vi "Linkages NodeID to GUID.vi"(7 "Response Refnum in":T1 format="%.0x", 8 "error in (no error)":errorcluster, 11 "Linked Channels in":T2[](array[typedef]) {"Channel Refnum" format="%.0x"}) -> (0 "error out":errorcluster, 3 "Linked Channels out":cluster{"Variable Name":string, "GUID":string}[](array[cluster]))   [LabVIEW 2018, in "Instrument Addon Scripting API.lvlib"]
uses:
  Instrument Addon Scripting API.lvlib
  TypeDefs/Linked Channel.ctl
  <vilib>/NI Veristand/Custom Device API/Custom Device Item Ref.ctl
  <vilib>/NI/NI VeriStand Advanced SysDef API/_SubVIs/SysDef.Search.Parent.vi
  Addon/Addon Shared/SubVIs/Constants.vi
  <vilib>/NI Veristand/Custom Device API/Get Item Property (String).vi
  <vilib>/NI Veristand/Custom Device API/Custom Device API.lvlib
  Addon/Addon Shared/Instrument Addon Shared.lvlib
  <vilib>/NI/NI VeriStand Advanced SysDef API/SysDef API/Advanced System Definition.lvlib
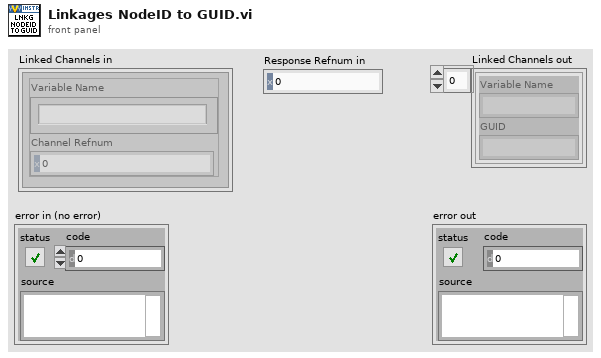
[diagram p1: front panel]
types:
  T1 = typedef "Custom Device API.lvlib/Custom Device Item Ref.ctl" = u64
  T2 = typedef "Instrument Addon Scripting API.lvlib/Linked Channel.ctl" = cluster{"Variable Name":string, "Channel Refnum":T1}
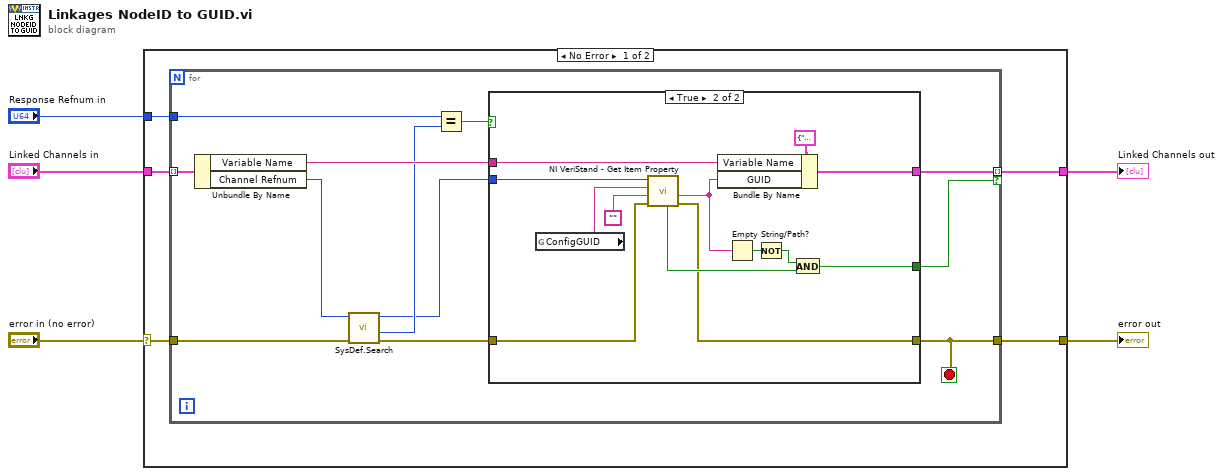
[diagram p0: block diagram]
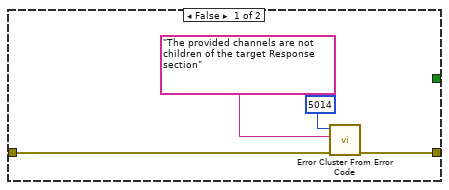
[diagram p2: hidden frame]
diagram:
  n1 = case shown="No Error" "error in (no error)" {
    selector: "error in (no error)" -> [w7 w40]
    tunnel: [w10 _] -> w5
    tunnel: [w9 w40] -> w4
    tunnel: "Linked Channels in" -> [w8 _]
    tunnel: "Response Refnum in" -> [w6 _]
    frame No Error {
      n2 = for {
        tunnel: w8 -> [w22] mode=indexing
        tunnel: w7 -> [w17]
        tunnel: [w20] -> w10 mode=indexing if=w19
        tunnel: [w18] -> w9
        tunnel: w6 -> [w14]
        stop <- w18 stop-if-true
        n3 = Unbundle By Name(w22) -> ("Variable Name"=w21:string, "Channel Refnum"=w16:T1)
        n4 = call-poly <vilib>:"SysDef.Search.vi"("error in (no error)"=w17, "nodeID"=w16) -> ("error out"=w13:errorcluster, "Value out"=w15:u64, "nodeID out"=w12:u64)  [unwired: 6 in, 1 out]
        n5 = Equal?(x=w14, y=w15) -> (x = y?=w11:bool)
        n6 = case shown="True" w11 {
          tunnel: w21 -> [_ w33]
          tunnel: [_ w31] -> w20
          tunnel: [_ w30] -> w19
          tunnel: [w25 w29] -> w18
          tunnel: w13 -> [w26 w28]
          tunnel: w12 -> [_ w27]
          frame False {
            n7 = call <vilib>:"Error Cluster From Error Code.vi"("error in (no error)"=w26, "error message (\"\")"="The provided channels are not children of the target Response section" ("error message (\"\")"), "error code (0)"=5014) -> ("error out"=w25:errorcluster)  [unwired: 6 in]
          }
          frame True {
            n8 = global read "Constants.vi" "ConfigGUID"() -> (w39:string)
            n9 = call-poly <vilib>:"NI VeriStand - Get Item Property.vi"("error in (no error)"=w28, "Default Value"="", "Property Name"=w39, "Item Ref in"=w27) -> ("error out"=w29:errorcluster, "Value"=w32:string, "Found?"=w37:bool)  [unwired: 4 in, 1 out]
            n10 = Bundle By Name(cluster=cluster{"Variable Name":string, "GUID":string} {"Variable Name"="", "GUID"=""}, "Variable Name"=w33, "GUID"=w32) -> (w31:cluster{"Variable Name":string, "GUID":string})
            n11 = Empty String/Path?(string/path=w32) -> (empty?=w36:bool)
            n12 = Not(x=w36) -> (.not. x?=w35:bool)
            n13 = And(x=w35, y=w37) -> (x .and. y?=w30:bool)
          }
        }
      }
    }
    frame Error {
    }
  }
  "Linked Channels out" <- w5
  "error out" <- w4
